vi "open.vi"(8 "error in (no error)":errorcluster, 11 "M1M3SAL in":refnum<class "M1M3SAL.lvclass">) -> (0 "error out":errorcluster, 3 "M1M3SAL out":refnum<class "M1M3SAL.lvclass">)   [LabVIEW 2016, in "M1M3SupportCommunicator.lvlib" / "M1M3SAL.lvclass"]
uses:
  M1M3SAL.lvclass
  M1M3SAL.lvclass/M1M3SAL.ctl
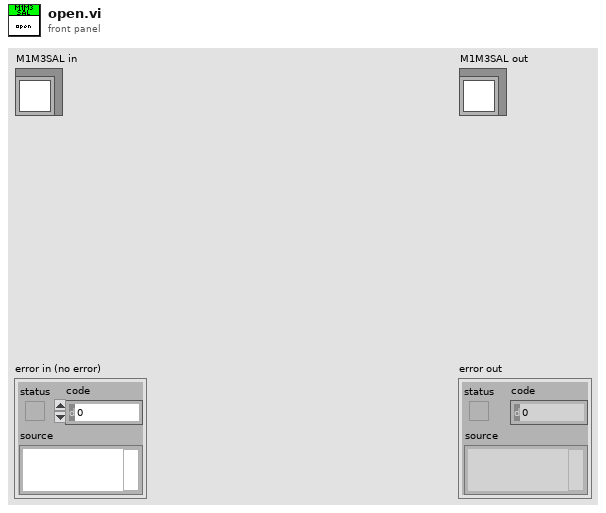
[diagram p1: front panel]
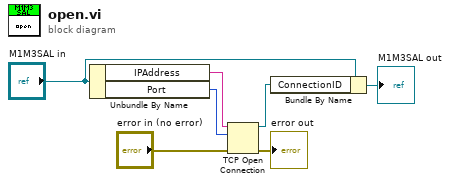
[diagram p0: block diagram]
diagram:
  n1 = Unbundle By Name("M1M3SAL in") -> ("IPAddress"=w7:string, "Port"=w6:u16)
  n2 = TCP Open Connection(address=w7, remote port or service name=w6, error in (no error)="error in (no error)") -> (connection ID=w4:refnum<k5>, error out=→"error out":errorcluster)  [unwired: 2 in]
  n3 = Bundle By Name(cluster="M1M3SAL in", "ConnectionID"=w4) -> (→"M1M3SAL out":refnum<class "M1M3SAL.lvclass">)
